vi "ProcessData.vi"(8 "error in (no error)":errorcluster, 9 "State":T1, 10 "Analog Data":T3, 11 "TwoAfcEye in":refnum<class "TwoAfcEye.lvclass">) -> (0 "error out":errorcluster, 1 "Fixated":bool, 2 "Trigger":T2=enum."Broke Fixation", 3 "TwoAfcEye out":refnum<class "TwoAfcEye.lvclass">)   [LabVIEW 2012, in "TwoAfcEye.lvclass"]
uses:
  TwoAfcEye.lvclass
  Core SubVIs/Controls/TYPE - Analog Data.ctl
  Trial Based Experiment Statechart/Trial Based Experiment.lvsc/Trigger.ctl
  Trial Based Experiment Statechart/Trial Based Experiment.lvsc/State.ctl
  <vilib>/measure/madcrms.llb/Basic Averaged DC-RMS for 1 Chan.vi
  Core SubVIs/Core SubVIs.lvlib
  <vilib>/measure/NI_MAPro.lvlib
  Trial Based Experiment Statechart/Trial Based Experiment.lvsc
  Acquisition/BehaviorData/BehaviorData.lvclass
panel:
  in  "Break Timeout (ms)":dbl
  in  "Adjustment Rate":dbl=0.02
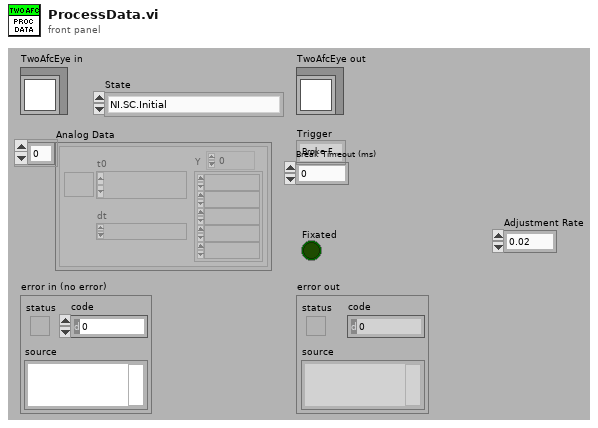
[diagram p1: front panel]
types:
  T1 = typedef "Trial Based Experiment.lvsc/State.ctl" = enum16{"NI.SC.Initial", "NI.SC.History", "NI.SC.ShallowHistory", "NI.SC.Terminal", "Cleanup", "State", "State\\Region\\Pause", "State\\Region\\Response Period", "State\\Region\\Delay Period", "State\\Region\\Hold Fixation", "State\\Region\\Acquire Fixation", "State\\Region\\Abort Trial", "State\\Region\\End Trial", "State\\Region\\Intertrial", "State\\Region\\Start Trial"}
  T2 = typedef "Trial Based Experiment.lvsc/Trigger.ctl" = enum16{"NULL", "Fixated", "Broke Fixation", "Stop", "Correct Response", "Incorrect Response", "Timeout"}
  T3 = typedef "Core SubVIs.lvlib/TYPE - Analog Data.ctl" = waveform(dbl)[]
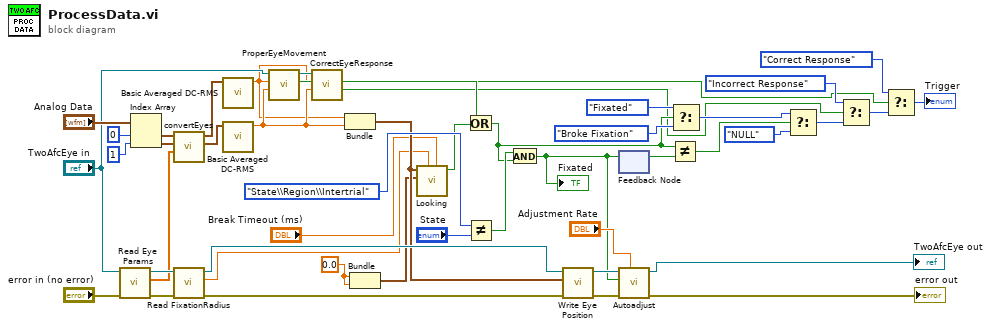
[diagram p0: block diagram]
diagram:
  w24 = 0.0
  n1 = call-dynamic "Read Eye Params.vi"("error in (no error)"="error in (no error)", "TrialBasedExperiment in"="TwoAfcEye in") -> ("error out"=w33:errorcluster, "Eye Params"=w41:dbl[], "TrialBasedExperiment out"=w47:refnum<class "TwoAfcEye.lvclass">)  [unwired: 7 in]
  n2 = Index Array(array="Analog Data", index #1=0 ("index"), index #2=1 ("index")) -> (element #1=w40:waveform(dbl), element #2=w39:waveform(dbl))
  n3 = call "convertEyes.vi"("Params"=w41, "Vertical"=w39, "Horizontal"=w40) -> ("Vertical Calibrated"=w44:waveform(dbl), "Horizontal Calibrated"=w43:waveform(dbl))  [unwired: 7 in]
  n4 = call-dynamic "Read FixationRadius.vi"("error in (no error)"=w33, "MatlabExperiment in"=w47) -> ("error out"=w29:errorcluster, "FixationRadius"=w22:dbl, "MatlabExperiment out"=w32:refnum<class "TwoAfcEye.lvclass">)  [unwired: 7 in]
  n5 = call-poly <vilib>:"Basic Averaged DC-RMS.vi"("signal in"=w43) -> ("DC value"=w1:dbl)  [unwired: 7 in, 3 out]
  n6 = call-poly <vilib>:"Basic Averaged DC-RMS.vi"("signal in"=w44) -> ("DC value"=w2:dbl)  [unwired: 7 in, 3 out]
  n7 = call-dynamic "ProperEyeMovement.vi"("y"=w2, "x"=w1, "TwoAfcEye in"="TwoAfcEye in") -> ("CorrectEye"=w13:bool, "TwoAfcEye out"=w10:refnum<class "TwoAfcEye.lvclass">)  [unwired: 6 in, 1 out]
  n8 = call-dynamic "CorrectEyeResponse.vi"("y"=w2, "x"=w1, "TwoAfcEye in"=w10) -> ("Incorrect Response"=w4:bool, "Correct Response"=w3:bool)  [unwired: 5 in, 2 out]
  n9 = Bundle("DC value"=w1, "DC value"=w2) -> (w25:cluster{"DC value":dbl, "DC value":dbl})  [unwired: 1 in]
  n10 = Bundle(w24, w24) -> (w23:cluster{dbl, dbl})  [unwired: 1 in]
  n11 = call "Looking.vi"("Break Timeout (ms)"="Break Timeout (ms)", "Fixation Radius (px)"=w22, "Desired Position"=w23, "Eye Position"=w25) -> ("Looking"=w12:bool)  [unwired: 6 in, 1 out]
  n12 = Or(x=w13, y=w12) -> (x .or. y?=w11:bool)
  n13 = Not Equal?(x=State."State\\Region\\Intertrial", y="State") -> (x != y?=w26:bool)
  n14 = And(x=w26, y=w11) -> (x .and. y?=w16:bool)
  "Fixated" <- w16
  n15 = call-dynamic "Write Eye Position.vi"("error in (no error)"=w29, "Eye Position"=w25, "TrialBasedExperiment in"=w32) -> ("error out"=w28:errorcluster, "TrialBasedExperiment out"=w31:refnum<class "TwoAfcEye.lvclass">)  [unwired: 7 in]
  n16 = feedback #1() -> (w36:bool)  [unwired: 1 in]
  n17 = feedback-in #1(w16) -> ()
  n18 = call-dynamic "Autoadjust.vi"("Adjustment Rate"="Adjustment Rate", "error in (no error)"=w28, "Fixated"=w16, "TrialBasedExperiment in"=w31) -> ("error out"=→"error out":errorcluster, "TrialBasedExperiment out"=→"TwoAfcEye out":refnum<class "TwoAfcEye.lvclass">)  [unwired: 6 in]
  n19 = Not Equal?(x=w11, y=w36) -> (x != y?=w34:bool)
  n20 = Select(t=Trigger."Fixated" ("Trigger"), s=w11, f=Trigger."Broke Fixation" ("Trigger")) -> (s? t:f=w37:T2)
  n21 = Select(t=w37, s=w34, f=Trigger."NULL" ("Trigger")) -> (s? t:f=w5:T2)
  n22 = Select(t=Trigger."Incorrect Response", s=w4, f=w5) -> (s? t:f=w9:T2)
  n23 = Select(t=Trigger."Correct Response", s=w3, f=w9) -> (s? t:f=→"Trigger":T2)
